vi "FormatLog.vi"(6 "log input":string, 8 "error in (no error)":errorcluster, 9 "System":string, 10 "Type":T1(ring), 11 "Log in":refnum<class "Log.lvclass">) -> (0 "error out":errorcluster, 3 "Log out":refnum<class "Log.lvclass">)   [LabVIEW 2018, in "Log.lvclass"]
uses:
  Log.lvclass
  Log.lvclass/Log.ctl
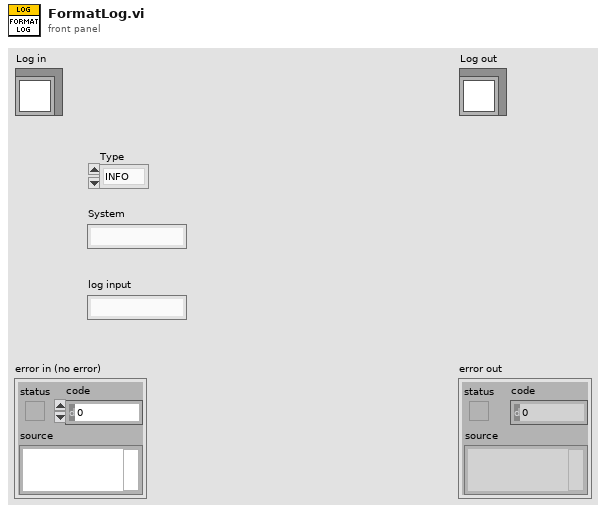
[diagram p1: front panel]
types:
  T1 = enum16{"INFO ", "TRACE", "DEBUG", "WARN ", "ERROR", "FATAL", "OTHER"}
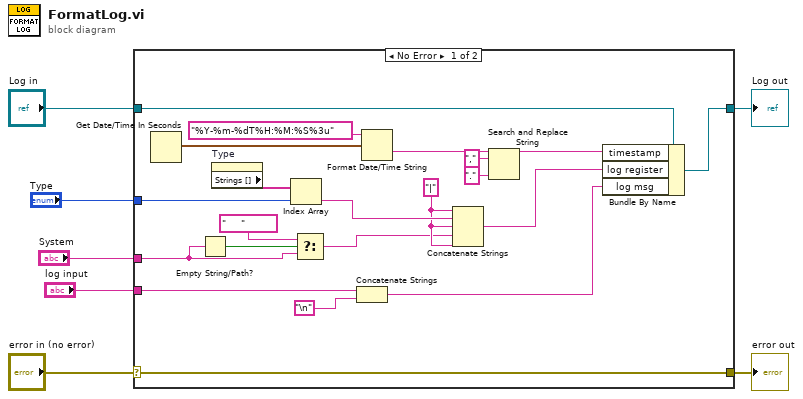
[diagram p0: block diagram]
diagram:
  n1 = case shown="No Error" "error in (no error)" {
    selector: "error in (no error)" -> [w28 w30]
    tunnel: [w28 w30] -> w6
    tunnel: [w19 w29] -> w4
    tunnel: "Log in" -> [w20 w29]
    tunnel: "Type" -> [w26 _]
    tunnel: "log input" -> [w11 _]
    tunnel: "System" -> [w15 _]
    frame No Error {
      w16 = "|" ("string")
      n2 = Get Date/Time In Seconds() -> (seconds since 1Jan1904=w24:timestamp)
      n3 = Empty String/Path?(string/path=w15) -> (empty?=w14:bool)
      n4 = property on="Type" class="Enum (strict)"() -> ("Strings []"=w27:string[])  [unwired: 2 in, 2 out]
      n5 = Index Array(array=w27, index=w26) -> (element=w17:string)
      n6 = Select(t="     ", s=w14, f=w15) -> (s? t:f=w13:string)
      n7 = Concatenate Strings(w11, "\n" ("string")) -> (w9:string)
      n8 = Format Date/Time String(time format string (%c)="%Y-%m-%dT%H:%M:%S%3u", seconds (now)=w24) -> (date/time string=w23:string)  [unwired: 1 in]
      n9 = Concatenate Strings(w16, w17, w16, w13, w16) -> (w12:string)
      n10 = Search and Replace String(input string=w23, search string=",", replace string="." ("replace string (\"\")")) -> (result string=w18:string)  [unwired: 5 in, 3 out]
      n11 = Bundle By Name(cluster=w20, "timestamp"=w18, "log register"=w12, "log msg"=w9) -> (w19:refnum<class "Log.lvclass">)
    }
    frame Error {
    }
  }
  "error out" <- w6
  "Log out" <- w4
